vi "PositionToReceivePass.vi"(8 "error in (no error)":errorcluster, 9 "Time Elapsed?":bool=TRUE, 10 "Game":refnum<class "Game.lvclass">, 11 "PositionToReceivePassSkill in":refnum<class "PositionToReceivePassSkill.lvclass">) -> (0 "error out":errorcluster, 2 "Position":dbl[](array[numeric]), 3 "PositionToReceivePassSkill out":refnum<class "PositionToReceivePassSkill.lvclass">)   [LabVIEW 2018, in "PositionToReceivePassSkill.lvclass"]
uses:
  PositionToReceivePassSkill.lvclass
  Game_class/Game.lvclass
  Game_class/Game.lvclass/Game.ctl
  Parameters_class/Parameters.lvclass/Parameters.ctl
  Game_class/Read Parameters.lvclass.vi
  Game_class/Read FieldRef.vi
  Parameters_class/Read AttakingOurselves.vi
  Parameters_class/Parameters.lvclass
  Field_class/Field.lvclass
  Utilities_class/Utilities.lvclass
  Ball_class/Ball.lvclass
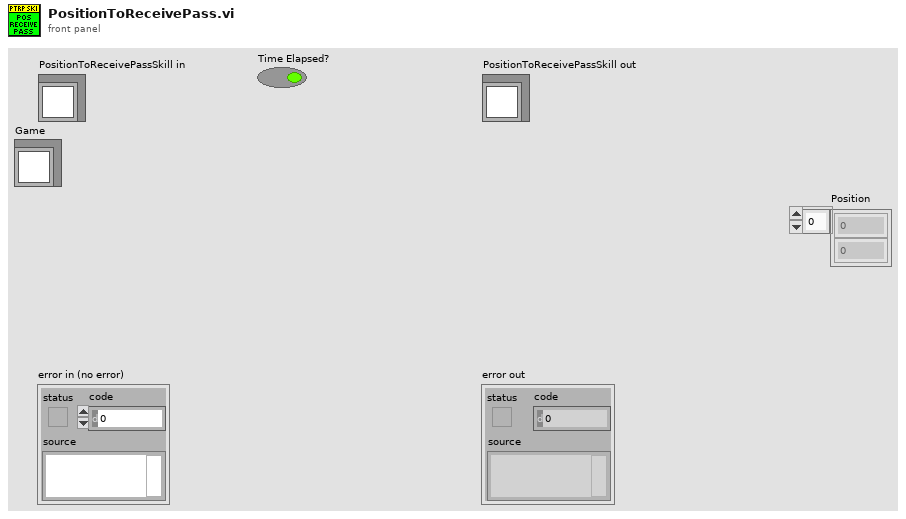
[diagram p1: front panel]
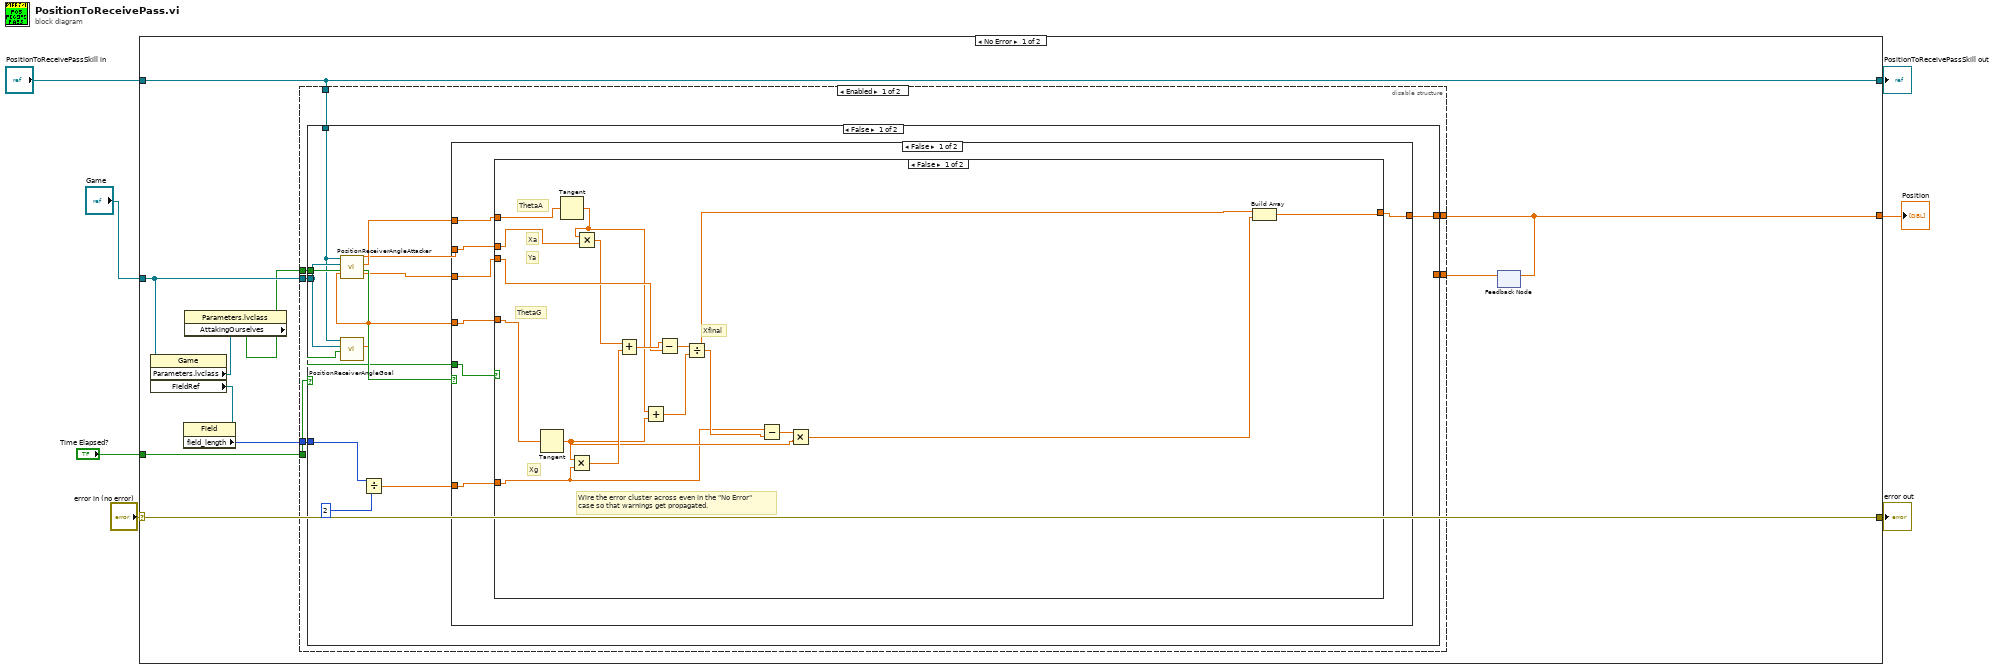
[diagram p0: block diagram]
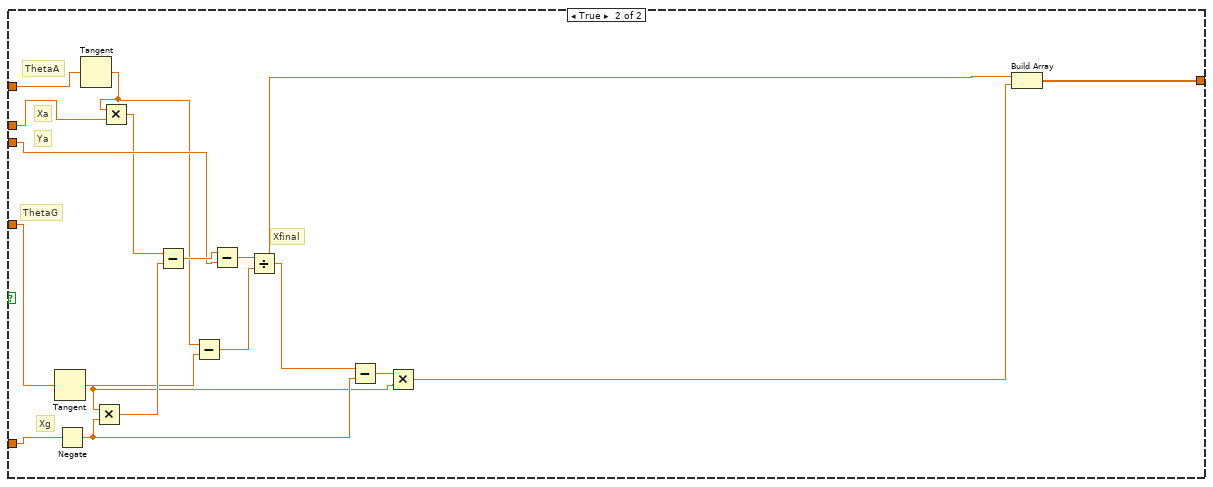
[diagram p2: hidden frame]
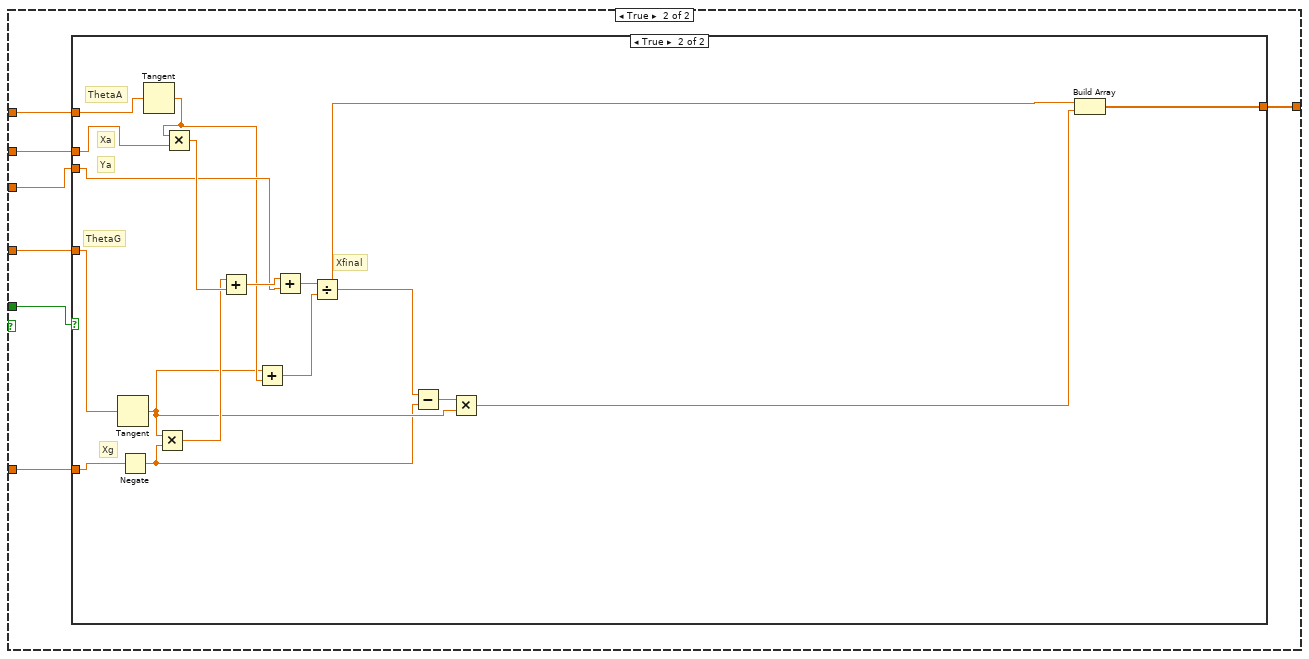
[diagram p3: hidden frame]
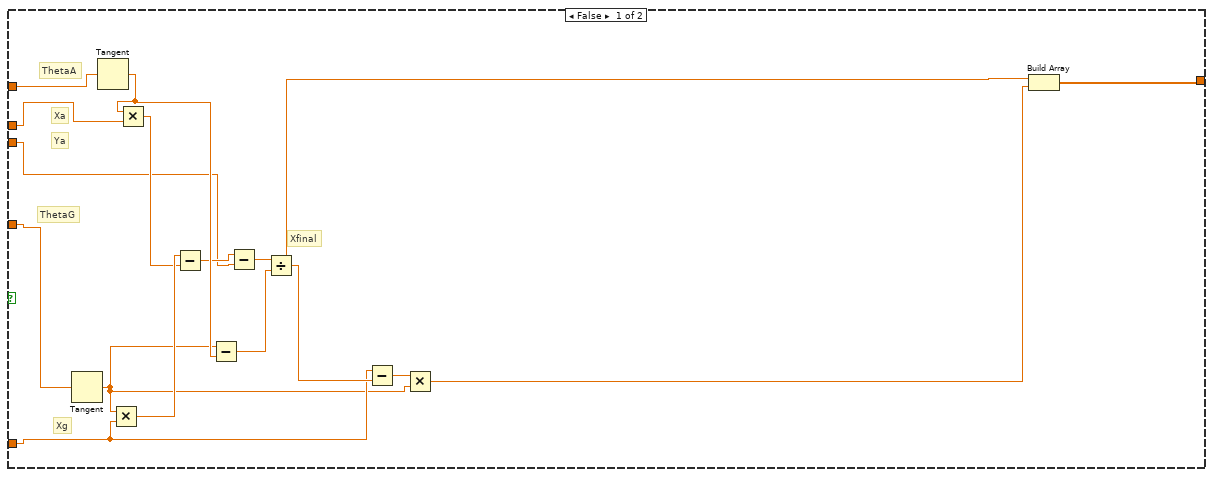
[diagram p4: hidden frame]
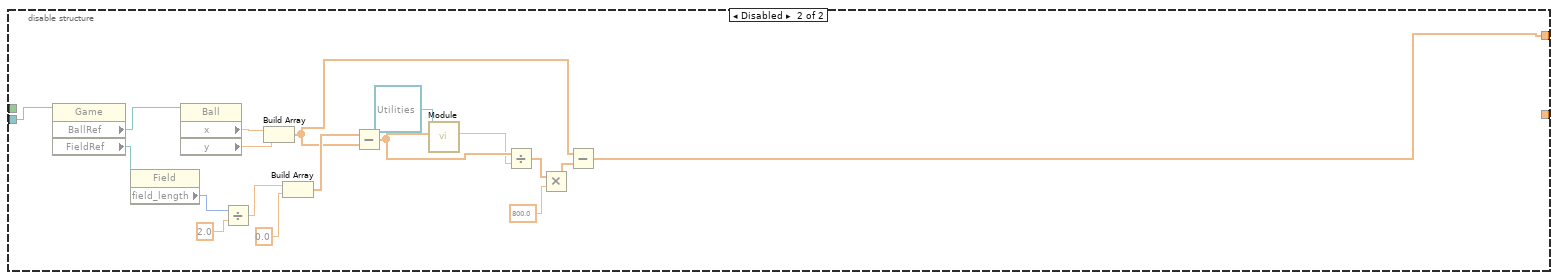
[diagram p6: hidden frame]
diagram:
  n1 = case shown="No Error" "error in (no error)" {
    selector: "error in (no error)" -> [w17 w137]
    tunnel: [w17 w137] -> w6
    tunnel: [w11 w136] -> w4
    tunnel: "PositionToReceivePassSkill in" -> [w11 w136]
    tunnel: "Game" -> [w13 _]
    tunnel: [w9 _] -> w2
    tunnel: "Time Elapsed?" -> [w10 _]
    frame No Error {
      n2 = property class="Game"(reference=w13) -> ("Parameters.lvclass"=w16:refnum<class "Parameters.lvclass">, "FieldRef"=w15:refnum<class "Field.lvclass">)  [unwired: 1 in, 2 out]
      n3 = property class="Field"(reference=w15) -> ("field_length"=w14:i32)  [unwired: 1 in, 2 out]
      n4 = property class="Parameters.lvclass"(reference=w16) -> ("AttakingOurselves"=w12:bool)  [unwired: 1 in, 2 out]
      n5 = feedback #1() -> (w8:dbl[])  [unwired: 1 in]
      n6 = disable-structure shown="Enabled" {
        disable-tunnel: w14 -> [w24 _]
        disable-tunnel: w13 -> [w23 w135]
        disable-tunnel: w12 -> [w22 _]
        disable-tunnel: w11 -> [w21 _]
        disable-tunnel: w10 -> [w20 _]
        disable-tunnel: [w19 w118] -> w9
        disable-tunnel: w8 -> [w18 _]
        frame Enabled {
          n7 = case shown="False" w20 {
            tunnel: w24 -> [w29 _]
            tunnel: w23 -> [w28 _]
            tunnel: w22 -> [w27 _]
            tunnel: w21 -> [w26 _]
            tunnel: [w25 w117] -> w19
            tunnel: w18 -> [_ w117]
            frame False {
              # "Wire the error cluster across even in the \"No Error\"\ncase so that warnings get propagated."
              n8 = call-dynamic "PositionReceiverAngleGoal.vi"("atacando contra"=w27, "Game"=w28, "PositionToReceivePassSkill in"=w26) -> ("theta final"=w30:dbl)  [unwired: 6 in, 2 out]
              n9 = call-dynamic "PositionReceiverAngleAttacker.vi"("AnguloGol"=w30, "atacando contra"=w27, "Game"=w28, "PositionToReceivePassSkill in"=w26) -> ("AttackerPositive?"=w36:bool, "theta final"=w35:dbl, "YdoAttacker 2"=w33:dbl, "XdoAttacker 2"=w34:dbl)  [unwired: 2 in, 2 out]
              n10 = Divide(x=w29, y=u32 2) -> (x/y=w31:dbl)
              n11 = case shown="False" w36 {
                tunnel: w27 -> [w37 w83]
                tunnel: w35 -> [w42 w82]
                tunnel: w34 -> [w41 w81]
                tunnel: w33 -> [w40 w80]
                tunnel: w30 -> [w39 w79]
                tunnel: w31 -> [w38 w78]
                tunnel: [w43 w77] -> w25
                frame False {
                  n12 = case shown="False" w37 {
                    tunnel: w42 -> [w53 w73]
                    tunnel: w41 -> [w52 w74]
                    tunnel: w40 -> [w51 w71]
                    tunnel: w39 -> [w54 w75]
                    tunnel: w38 -> [w44 w76]
                    tunnel: [w50 w66] -> w43
                    frame False {
                      # "Xfinal"
                      # "Xg"
                      # "ThetaG"
                      # "Ya"
                      # "Xa"
                      # "ThetaA"
                      n13 = Tangent(1:w54) -> (0:w46:dbl)
                      n14 = Tangent(1:w53) -> (0:w47:dbl)
                      n15 = Multiply(x=w46, y=w44) -> (x*y=w49:dbl)
                      n16 = Multiply(x=w47, y=w52) -> (x*y=w48:dbl)
                      n17 = Add(x=w48, y=w49) -> (x+y=w55:dbl)
                      n18 = Add(x=w47, y=w46) -> (x+y=w57:dbl)
                      n19 = Subtract(x=w55, y=w51) -> (x-y=w56:dbl)
                      n20 = Divide(x=w56, y=w57) -> (x/y=w45:dbl)
                      n21 = Subtract(x=w44, y=w45) -> (x-y=w58:dbl)
                      n22 = Multiply(x=w58, y=w46) -> (x*y=w59:dbl)
                      n23 = Build Array(w45, w59) -> (w50:dbl[])
                    }
                    frame True {
                      # "Xfinal"
                      # "Xg"
                      # "ThetaG"
                      # "Ya"
                      # "Xa"
                      # "ThetaA"
                      n24 = Tangent(1:w75) -> (0:w60:dbl)
                      n25 = Negate(x=w76) -> (-x=w65:dbl)
                      n26 = Tangent(1:w73) -> (0:w61:dbl)
                      n27 = Multiply(x=w60, y=w65) -> (x*y=w63:dbl)
                      n28 = Multiply(x=w61, y=w74) -> (x*y=w62:dbl)
                      n29 = Subtract(x=w62, y=w63) -> (x-y=w72:dbl)
                      n30 = Subtract(x=w61, y=w60) -> (x-y=w69:dbl)
                      n31 = Subtract(x=w72, y=w71) -> (x-y=w70:dbl)
                      n32 = Divide(x=w70, y=w69) -> (x/y=w64:dbl)
                      n33 = Subtract(x=w64, y=w65) -> (x-y=w68:dbl)
                      n34 = Multiply(x=w68, y=w60) -> (x*y=w67:dbl)
                      n35 = Build Array(w64, w67) -> (w66:dbl[])
                    }
                  }
                }
                frame True {
                  n36 = case shown="True" w83 {
                    tunnel: w82 -> [w89 w113]
                    tunnel: w81 -> [w88 w114]
                    tunnel: w80 -> [w87 w109]
                    tunnel: w79 -> [w90 w115]
                    tunnel: w78 -> [w86 w116]
                    tunnel: [w85 w104] -> w77
                    frame False {
                      # "Xfinal"
                      # "Xg"
                      # "ThetaG"
                      # "Ya"
                      # "Xa"
                      # "ThetaA"
                      n37 = Tangent(1:w90) -> (0:w84:dbl)
                      n38 = Tangent(1:w89) -> (0:w98:dbl)
                      n39 = Multiply(x=w84, y=w86) -> (x*y=w92:dbl)
                      n40 = Multiply(x=w98, y=w88) -> (x*y=w91:dbl)
                      n41 = Subtract(x=w92, y=w91) -> (x-y=w93:dbl)
                      n42 = Subtract(x=w84, y=w98) -> (x-y=w95:dbl)
                      n43 = Subtract(x=w93, y=w87) -> (x-y=w94:dbl)
                      n44 = Divide(x=w94, y=w95) -> (x/y=w96:dbl)
                      n45 = Subtract(x=w86, y=w96) -> (x-y=w97:dbl)
                      n46 = Multiply(x=w97, y=w84) -> (x*y=w99:dbl)
                      n47 = Build Array(w96, w99) -> (w85:dbl[])
                    }
                    frame True {
                      # "Xfinal"
                      # "Xg"
                      # "ThetaG"
                      # "Ya"
                      # "Xa"
                      # "ThetaA"
                      n48 = Tangent(1:w115) -> (0:w102:dbl)
                      n49 = Negate(x=w116) -> (-x=w101:dbl)
                      n50 = Tangent(1:w113) -> (0:w103:dbl)
                      n51 = Multiply(x=w102, y=w101) -> (x*y=w111:dbl)
                      n52 = Multiply(x=w103, y=w114) -> (x*y=w112:dbl)
                      n53 = Add(x=w111, y=w112) -> (x+y=w110:dbl)
                      n54 = Add(x=w102, y=w103) -> (x+y=w107:dbl)
                      n55 = Add(x=w110, y=w109) -> (x+y=w108:dbl)
                      n56 = Divide(x=w108, y=w107) -> (x/y=w100:dbl)
                      n57 = Subtract(x=w100, y=w101) -> (x-y=w106:dbl)
                      n58 = Multiply(x=w106, y=w102) -> (x*y=w105:dbl)
                      n59 = Build Array(w100, w105) -> (w104:dbl[])
                    }
                  }
                }
              }
            }
            frame True {
            }
          }
        }
        frame Disabled {
          n60 = property class="Game"(reference=w135) -> ("BallRef"=w134:refnum<class "Ball.lvclass">, "FieldRef"=w133:refnum<class "Field.lvclass">)  [unwired: 1 in, 2 out]
          n61 = property class="Field"(reference=w133) -> ("field_length"=w130:i32)  [unwired: 1 in, 2 out]
          n62 = property class="Ball"(reference=w134) -> ("x"=w132:dbl, "y"=w131:dbl)  [unwired: 1 in, 2 out]
          n63 = Divide(x=w130, y=2.0) -> (x/y=w128:dbl)
          n64 = Build Array(w132, w131) -> (w122:dbl[])
          n65 = Build Array(w128, 0.0) -> (w126:dbl[])
          n66 = Subtract(x=w126, y=w122) -> (x-y=w124:dbl[])
          n67 = call-dynamic "Module.vi"("2D vector"=w124, "Utilities in"=refnum<class "Utilities.lvclass"> refnum) -> ("Modulo"=w123:dbl)  [unwired: 7 in, 2 out]
          n68 = Divide(x=w124, y=w123) -> (x/y=w121:dbl[])
          n69 = Multiply(x=w121, y=800.0) -> (x*y=w119:dbl[])
          n70 = Subtract(x=w122, y=w119) -> (x-y=w118:dbl[])
        }
      }
      n71 = feedback-in #1(w9) -> ()
    }
    frame Error {
    }
  }
  "error out" <- w6
  "PositionToReceivePassSkill out" <- w4
  "Position" <- w2
